vi "Read Rig Config Info.vi"(11 "Rig File Name":string) -> ()   [LabVIEW 2018]
uses:
  controls/Rig Config Settings.ctl
  controls/Command IN_Recipe.ctl
  Globals/Global - Configuration Options.vi
panel:
  out "Rig Config Settings":T1={"Rig Name"="", "Rig Room"="", "Base Directory"="", "Computer IP Address"="", "Globals Name"="", "Treatmill Str"="", "Data Dir"="", "ai"="", "ao"="", "dio"="", "A_calib_str_row1"="", "A_calib_str_row2"="", "A_calib_str_row3"="", "Zero_V_str"="", "step_V"="", "Sample Freq"="", "ai_threshold"="", "run_speed_thresh"="", "speed_time_length"="", "wall ball gain"="", "max wall pos"="", "max cor width"="", "Rig Config Directory"=path "C:/Whisker Tester/Rig", "Trial Config Directory"=path "C:/Whisker Tester/Trials"}
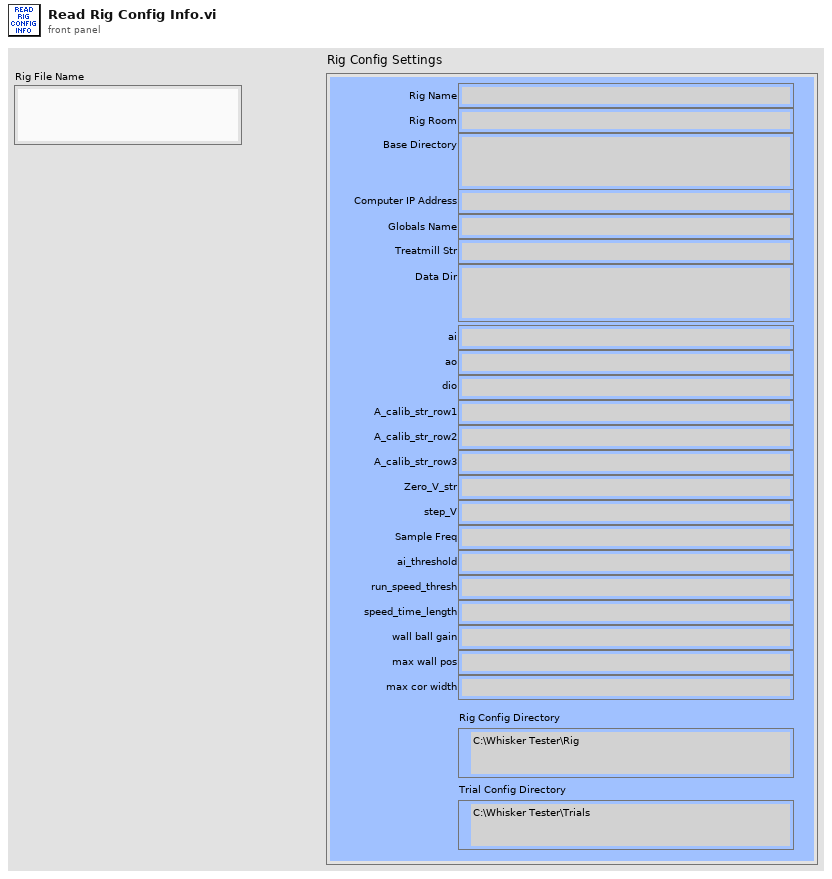
[diagram p1: front panel]
types:
  T1 = typedef "Rig Config Settings.ctl" = cluster{"Rig Name":string, "Rig Room":string, "Base Directory":string, "Computer IP Address":string, "Globals Name":string, "Treatmill Str":string, "Data Dir":string, "ai":string, "ao":string, "dio":string, "A_calib_str_row1":string, "A_calib_str_row2":string, "A_calib_str_row3":string, "Zero_V_str":string, "step_V":string, "Sample Freq":string, "ai_threshold":string, "run_speed_thresh":string, "speed_time_length":string, "wall ball gain":string, "max wall pos":string, "max cor width":string, "Rig Config Directory":path, "Trial Config Directory":path}
  T2 = typedef "Command IN_Recipe.ctl" = enum16{"Save", "Load"}
  T3 = typedef "Labview Settings.ctl" = cluster{"Rig Config Directory":path, "Trial Config Directory":path, "Computer IP Address":string, "cRIO IP Address":string}
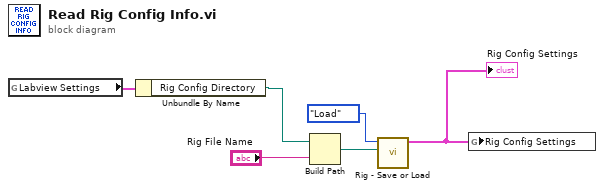
[diagram p0: block diagram]
diagram:
  n1 = global read "Global - Configuration Options.vi" "Labview Settings"() -> (w5:T3)
  n2 = Unbundle By Name(w5) -> ("Rig Config Directory"=w4:path)
  n3 = Build Path(base path=w4, name or relative path="Rig File Name") -> (appended path=w2:path)
  n4 = call "Rig - Save or Load.vi"("RigSave Path IN"=w2, "Command IN"=Command_IN_Recipe."Load") -> ("Rig Settings OUT"=w1:T1)  [unwired: 8 in, 1 out]
  "Rig Config Settings" <- w1
  n5 = global write "Global - Configuration Options.vi" "Rig Config Settings"(w1) -> ()
